vi "Destroy.vi"(0 "reference in":refnum<class "IG#InterfaceTemplate.lvclass">, 5 "error in (no error)":errorcluster) -> (14 "reference out":refnum<class "IG#InterfaceTemplate.lvclass">, 19 "error out":errorcluster)   [LabVIEW 2020, in "IG#InterfaceTemplate.lvclass"]
doc: "G#Object destructor."
uses:
  IG#InterfaceTemplate.lvclass
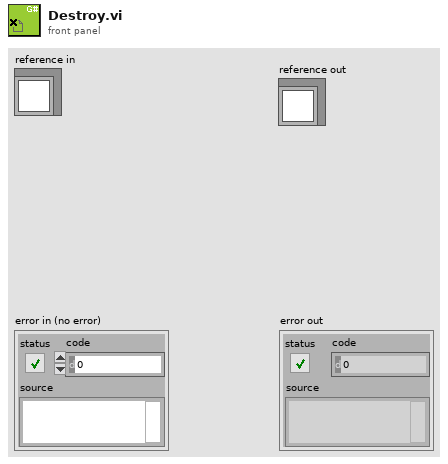
[diagram p1: front panel]
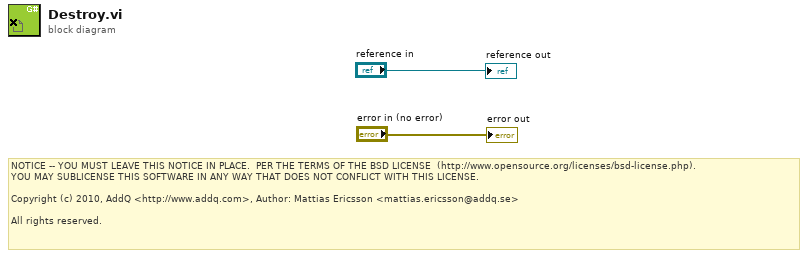
[diagram p0: block diagram]
diagram:
  # "NOTICE -- YOU MUST LEAVE THIS NOTICE IN PLACE.  PER THE TERMS OF THE BSD LICENSE  (http://www.opensource.org/licenses/bsd-license.php).\nYOU MAY SUBLICENSE THIS SOFTWARE IN ANY WAY THAT DOES NOT CONFLICT WITH THIS LICENSE.\n\nCopyright (c) 2010, AddQ <http://www.addq.com>, Author: Mattias Ericsson <mattias.ericsson@addq.se>\n\nAll rights reserved."
  "error out" <- "error in (no error)"
  "reference out" <- "reference in"
